vi "Read Independent Variables.vi"(8 "error in (no error)":errorcluster, 11 "Double Scanner.lvclass in":refnum<class "Double Scanner.lvclass">) -> (0 "error out":errorcluster, 1 "size":i32, 2 "Independent Variables":dbl[][](array[numeric]), 3 "Double Scanner.lvclass out":refnum<class "Double Scanner.lvclass">, 4 "min value":dbl, 5 "max value":dbl)   [LabVIEW 2012, in "Double Scanner.lvclass"]
doc: "Return the internal array of independent variables for this Scanner, e.g., to write out to a file. Use this method with extreme caution, since it breaks the encapsulation for this class. Do not use it to manipulate a Scanner's internal state."
uses:
  Double Scanner.lvclass
  Scanner/Scanner.lvclass
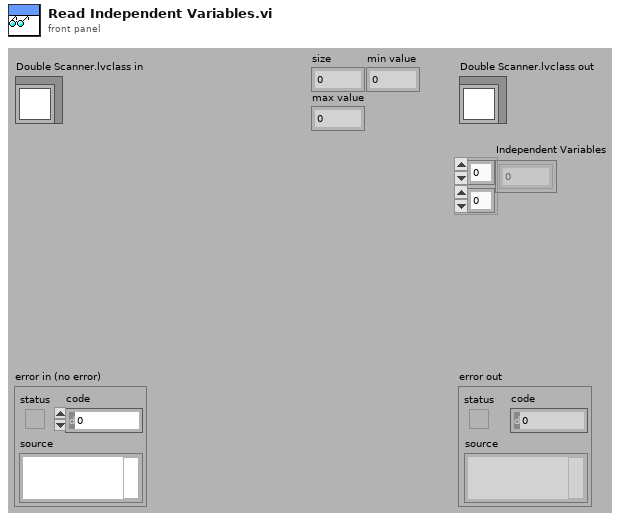
[diagram p1: front panel]
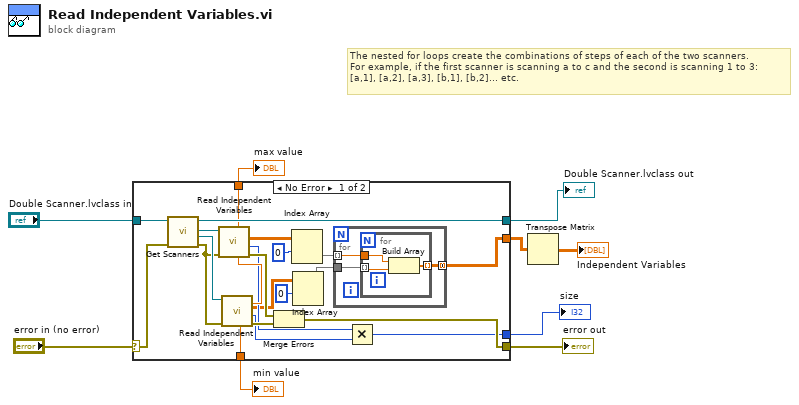
[diagram p0: block diagram]
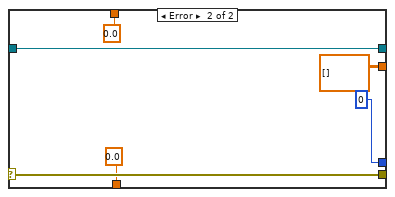
[diagram p2: hidden frame]
diagram:
  # "The nested for loops create the combinations of steps of each of the two scanners.\nFor example, if the first scanner is scanning a to c and the second is scanning 1 to 3:\n[a,1], [a,2], [a,3], [b,1], [b,2]... etc."
  n1 = case shown="No Error" "error in (no error)" {
    selector: "error in (no error)" -> [w28 w41]
    tunnel: [w22 w41] -> w8
    tunnel: "Double Scanner.lvclass in" -> [w30 w42]
    tunnel: [w29 w42] -> w6
    tunnel: [w10 dbl[][] []] -> w2
    tunnel: [w21 0.0 ("max value")] -> w5
    tunnel: [w20 0.0 ("min value")] -> w4
    tunnel: [w17 0] -> w3
    frame No Error {
      n2 = call-dynamic "Get Scanners.vi"("error in (no error)"=w28, "Double Scanner in"=w30) -> ("error out"=w25:errorcluster, "Scanner 2 out"=w26:refnum<class "Scanner.lvclass">, "Scanner 1 out"=w27:refnum<class "Scanner.lvclass">, "Double Scanner out"=w29:refnum<class "Double Scanner.lvclass">)  [unwired: 6 in]
      n3 = call-dynamic "Read Independent Variables.vi"("error in (no error)"=w25, "Scanner.lvclass in"=w27) -> ("error out"=w24:errorcluster, "size"=w19:i32, "Independent Variables"=w15:dbl[][], "min value"=w20:dbl, "max value"=w21:dbl)  [unwired: 4 in, 1 out]
      n4 = call-dynamic "Read Independent Variables.vi"("error in (no error)"=w25, "Scanner.lvclass in"=w26) -> ("error out"=w23:errorcluster, "size"=w18:i32, "Independent Variables"=w16:dbl[][])  [unwired: 4 in, 3 out]
      n5 = Merge Errors(w24, w23) -> (w22:errorcluster)
      n6 = Index Array(array=w15, index (row)=0) -> (element=w12:dbl[])  [unwired: 1 in]
      n7 = Index Array(array=w16, index (row)=0) -> (element=w11:dbl[])  [unwired: 1 in]
      n8 = for {
        tunnel: w12 -> [w32] mode=indexing
        tunnel: w11 -> [w33]
        tunnel: [w31] -> w10 mode=concatenating
        n9 = for {
          tunnel: w33 -> [w35] mode=indexing
          tunnel: w32 -> [w36]
          tunnel: [w34] -> w31 mode=indexing
          n10 = Build Array(w36, w35) -> (w34:dbl[])
        }
      }
      n11 = Multiply(x=w19, y=w18) -> (x*y=w17:i32)
    }
    frame Error {
    }
  }
  "error out" <- w8
  "Double Scanner.lvclass out" <- w6
  "size" <- w3
  "min value" <- w4
  "max value" <- w5
  n12 = Transpose Matrix(1:w2) -> (0:→"Independent Variables":dbl[][])
